vi "Set Order Queue Handler.vi"(8 "error in (no error)":errorcluster, 10 "Order Queue Handler":refnum<class "Job Handler.lvclass">, 11 "Coffee Shop In":refnum<class "Coffee Shop.lvclass">) -> (0 "error out":errorcluster, 3 "Coffee Shop Out":refnum<class "Coffee Shop.lvclass">)   [LabVIEW 2020, in "Coffee Shop.lvclass"]
uses:
  Coffee Shop.lvclass
  C:/Program Files (x86)/National Instruments/LabVIEW 2020/vi.lib/Astemes/Triarc Framework/Process/Process.lvclass
  C:/Program Files (x86)/National Instruments/LabVIEW 2020/vi.lib/Astemes/Triarc Framework/Application/Application.lvclass
  People/Process Job/Job Handler.lvclass
  <vilib>/Astemes/Triarc Framework/Process/Process.lvclass
  <vilib>/Astemes/Triarc Framework/Process/Process.lvclass/Process.ctl
  <vilib>/Astemes/Triarc Framework/Process/Private/SubVIs/Handle Debug Data.vi
  <vilib>/Astemes/Triarc Framework/Logging/Log Debug.vi
  <vilib>/AdvancedString/1D String Array to Delimited String.vi
  <vilib>/Utility/High Resolution Relative Seconds.vi
  <vilib>/Astemes/Triarc Framework/Process/Public/Read Name.vi
  <vilib>/Astemes/Triarc Framework/Callback/Callback.lvclass
  <vilib>/Astemes/Triarc Framework/Application/Application.lvclass
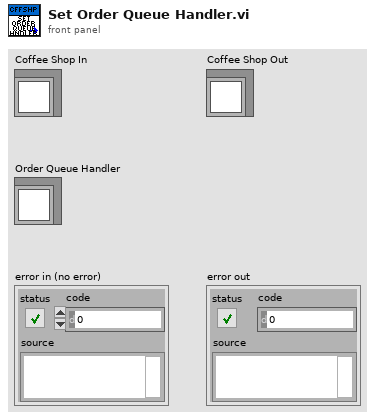
[diagram p1: front panel]
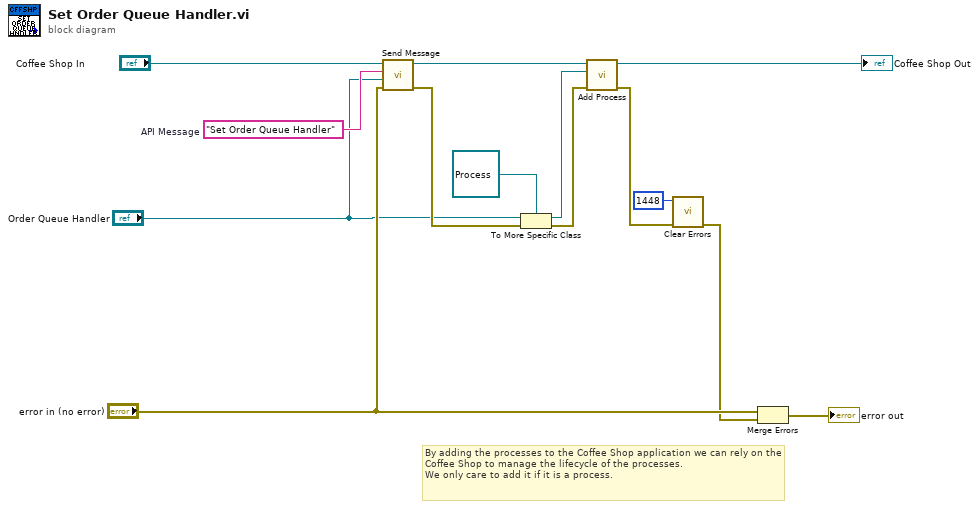
[diagram p0: block diagram]
diagram:
  w2 = "Set Order Queue Handler"  # API Message
  # "By adding the processes to the Coffee Shop application we can rely on the Coffee Shop to manage the lifecycle of the processes.\nWe only care to add it if it is a process."
  n1 = call <vilib>:"Send Message.vi"("error in (no error)"="error in (no error)", "Message Data"="Order Queue Handler", "Message"=w2, "Process In"="Coffee Shop In") -> ("error out"=w5:errorcluster, "Process Out"=w10:refnum<class "Coffee Shop.lvclass">)  [unwired: 6 in]
  n2 = To More Specific Class(target class=refnum<class "Process.lvclass"> refnum ("Process Out"), reference="Order Queue Handler", error in=w5) -> (specific class reference=w8:refnum<class "Process.lvclass">, error out=w6:errorcluster)
  n3 = call <vilib>:"Add Process.vi"("error in (no error)"=w6, "Process"=w8, "Application In"=w10) -> ("error out"=w9:errorcluster, "Application Out"=→"Coffee Shop Out":refnum<class "Coffee Shop.lvclass">)  [unwired: 7 in]
  n4 = call <vilib>:"Clear Errors.vi"("error in (no error)"=w9, "specific error code to clear (0: all)"=1448) -> ("error out"=w4:errorcluster)  [unwired: 4 in, 1 out]
  n5 = Merge Errors("error in (no error)", w4) -> (→"error out":errorcluster)
